vi "Register For Events.vi"(8 "error in":errorcluster, 10 "Table Events":T1, 11 "References":T2) -> (0 "error out":errorcluster, 3 "Event Registration Refnum":refnum<event-registration>)   [LabVIEW 2018, in "Benchmark PID editor node.lvclass"]
doc: "In this VI we register the events that will be handled by the Node UI. We need to include the ones we are interested in handling from the Configuration editor as well as the ones from the table."
uses:
  Benchmark PID editor node.lvclass
  <vilib>/NI/DCAF/Tag Editor Core/Table API/Table Manager/references.ctl
  <vilib>/NI/Configuration Framework/Node/StopEvent.ctl
  <vilib>/NI/Configuration Framework/Node/RefreshUIEvent.ctl
  <vilib>/NI/Configuration Framework/Node/CacheState.ctl
  <vilib>/NI/Configuration Framework/Node/NodeChangeEvent.ctl
  <vilib>/NI/Configuration Framework/Node/NodeRef.ctl
  <vilib>/NI/Configuration Framework/Node/NISE_CEF_Node.lvclass
  <vilib>/NI/DCAF/Tag Editor Core/Table API/Available Tag Menu/channel action event.ctl
  <vilib>/NI/DCAF/Tag Editor Core/Table API/Available Tag Menu/dialog output action.ctl
  <vilib>/NI/Tag Bus Module Framework/channel/TBM channel.lvclass
  <vilib>/NI/Tag Bus/tag/tag descriptor.lvclass
  <vilib>/NI/DCAF/Tag Editor Core/Table API/Table Manager/Call Back Ref Type Def.ctl
  <vilib>/NI/DCAF/Tag Editor Core/Configuration Editor/Classes/Engine Parent/Engine Parent Editor Node.lvclass
  <vilib>/NI/DCAF/Tag Editor Core/Configuration Editor/Classes/Module editor node/module editor node.lvclass
  <vilib>/NI/AMC/Message Queue.ctl
  <vilib>/NI/AMC/Message.ctl
  <vilib>/NI/Tools/Keyed Array/KeyedArray.ctl
  <vilib>/NI/Configuration Framework/Node/UserEventRef.ctl
  <vilib>/NI/Configuration Framework/Controls/EventCluster.ctl
  <vilib>/NI/DCAF/Tag Editor Core/Table API/Table Manager/Table Events.ctl
  <vilib>/NI/DCAF/Tag Editor Core/Table API/Table Manager/Menu Select.ctl
  <vilib>/NI/Configuration Framework/NISE_CEF_TreeControl.lvlib
  <vilib>/NI/DCAF/Tag Editor Core/Table API/Table Manager.lvlib
  <vilib>/NI/Tools/Keyed Array/Tools_KeyedArray.lvlib
  <vilib>/NI/AMC/AMC.lvlib
  <vilib>/NI/DCAF/Tag Editor Core/Table API/Table Manager/Table Manager.lvclass
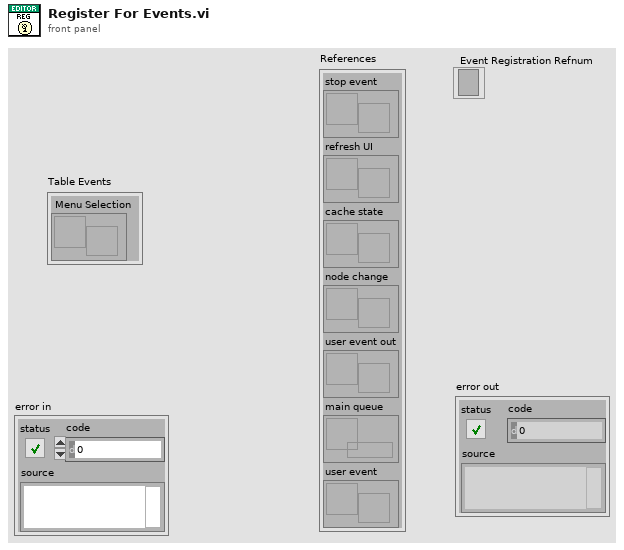
[diagram p1: front panel]
types:
  T1 = typedef "Table Manager.lvlib/Table Manager.lvclass/Table Events.ctl" = cluster{"Menu Selection":refnum<user-event>}
  T2 = typedef "Table Manager.lvlib/Table Manager.lvclass/references.ctl" = cluster{"stop event":T3, "refresh UI":T4, "cache state":T5, "node change":T6, "user event out":refnum<user-event>, "main queue":T7, "user event":T8}
  T3 = typedef "NISE_CEF_Node.lvclass/StopEvent.ctl" = refnum<user-event>
  T4 = typedef "NISE_CEF_Node.lvclass/RefreshUIEvent.ctl" = refnum<user-event>
  T5 = typedef "NISE_CEF_Node.lvclass/CacheState.ctl" = refnum<user-event>
  T6 = typedef "NISE_CEF_Node.lvclass/NodeChangeEvent.ctl" = refnum<user-event>
  T7 = typedef "AMC.lvlib/Message Queue.ctl" = refnum<queue>
  T8 = typedef "NISE_CEF_Node.lvclass/UserEventRef.ctl" = refnum<user-event>
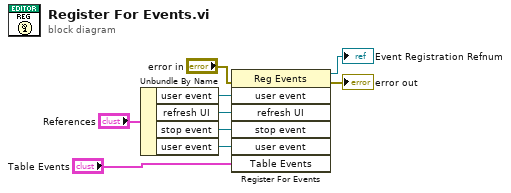
[diagram p0: block diagram]
diagram:
  n1 = Unbundle By Name("References") -> ("user event"=w7:T8, "refresh UI"=w6:T4, "stop event"=w5:T3, "user event"=w4:T8)
  n2 = register-events(error in="error in", w7, w6, w5, w4, "Table Events") -> (reference out=→"Event Registration Refnum":refnum<event-registration>, error out=→"error out":errorcluster)  [unwired: 1 in]
